vi "MGCC_StaEst_initial_3.vi"() -> ()   [LabVIEW 2016]
uses:
  <vilib>/imath/engines/lvmath2/RunTimeEngine/RunTimeType/NIMS_RunTimeType_From StrictType (excl LVString).vi
  <instcachedir>/0/NIMS_RunTimeType_From StrictType (excl LVString)_BBF44FB49F834B71AF7A14CCEDF8BECD.lvgen/NIMS_RunTimeType_From StrictType (excl LVString)_BBF44FB49F834B71AF7A14CCEDF8BECD_032.vi
  <instcachedir>/0/NIMS_RunTimeType_From StrictType (excl LVString)_BBF44FB49F834B71AF7A14CCEDF8BECD.lvgen/NIMS_RunTimeType_From StrictType (excl LVString)_BBF44FB49F834B71AF7A14CCEDF8BECD_031.vi
  <vilib>/imath/engines/lvmath2/RunTimeEngine/Struct/NIMS_StructSetField.vi
  <vilib>/imath/engines/lvmath2/RunTimeEngine/Struct/NIMS_StructGetField.vi
  <vilib>/imath/engines/lvmath2/RunTimeEngine/RunTimeType/NIMS_RunTimeType_To Numeric.vi
  <instcachedir>/0/NIMS_RunTimeType_To Numeric_19D51BCABB82435A94073491761E42EE.lvgen/NIMS_RunTimeType_To Numeric_19D51BCABB82435A94073491761E42EE_009.vi
  <vilib>/imath/engines/lvmath2/RunTimeEngine/RangeToken/NIMS_Range.vi
  <instcachedir>/0/NIMS_Range_A7C094595B484CA7AF10685B02D808ED.lvgen/NIMS_Range_A7C094595B484CA7AF10685B02D808ED_000.vi
  <instcachedir>/0/NIMS_RunTimeType_From StrictType (excl LVString)_BBF44FB49F834B71AF7A14CCEDF8BECD.lvgen/NIMS_RunTimeType_From StrictType (excl LVString)_BBF44FB49F834B71AF7A14CCEDF8BECD_010.vi
  <vilib>/imathl/engines/lvmath/Functions/Error Handling/Create Error.vi
  <instcachedir>/0/NIMS_RunTimeType_To Numeric_19D51BCABB82435A94073491761E42EE.lvgen/NIMS_RunTimeType_To Numeric_19D51BCABB82435A94073491761E42EE_004.vi
  <instcachedir>/0/NIMS_RunTimeType_From StrictType (excl LVString)_BBF44FB49F834B71AF7A14CCEDF8BECD.lvgen/NIMS_RunTimeType_From StrictType (excl LVString)_BBF44FB49F834B71AF7A14CCEDF8BECD_024.vi
  <instcachedir>/0/NIMS_RunTimeType_To Numeric_19D51BCABB82435A94073491761E42EE.lvgen/NIMS_RunTimeType_To Numeric_19D51BCABB82435A94073491761E42EE_008.vi
  <vilib>/imath/engines/lvmath2/RunTimeEngine/NodeEndStatement/NIMS_NodeEndStatement_Output.vi
  <instcachedir>/0/NIMS_NodeEndStatement_Output_53EC0D466D134D7ABD903AC30B43404B.lvgen/NIMS_NodeEndStatement_Output_53EC0D466D134D7ABD903AC30B43404B_001.vi
  <instcachedir>/0/NIMS_NodeEndStatement_Output_53EC0D466D134D7ABD903AC30B43404B.lvgen/NIMS_NodeEndStatement_Output_53EC0D466D134D7ABD903AC30B43404B_011.vi
  <instcachedir>/0/NIMS_NodeEndStatement_Output_53EC0D466D134D7ABD903AC30B43404B.lvgen/NIMS_NodeEndStatement_Output_53EC0D466D134D7ABD903AC30B43404B_023.vi
  <instcachedir>/0/NIMS_NodeEndStatement_Output_53EC0D466D134D7ABD903AC30B43404B.lvgen/NIMS_NodeEndStatement_Output_53EC0D466D134D7ABD903AC30B43404B_029.vi
  <instcachedir>/0/NIMS_NodeEndStatement_Output_53EC0D466D134D7ABD903AC30B43404B.lvgen/NIMS_NodeEndStatement_Output_53EC0D466D134D7ABD903AC30B43404B_019.vi
  <vilib>/imath/engines/lvmath2/RunTimeEngine/ErrorHandling/NIMS_Finalize Error.vi
panel:
  out "iterMax":i32
  out "tol":dbl
  out "MeaIdx":cluster{"PN":dbl[], "QN":dbl[], "VN":dbl[]}
  out "MeaPha":T1
  out "interleaved array":dbl[](array[numeric])
  out "error out":errorcluster
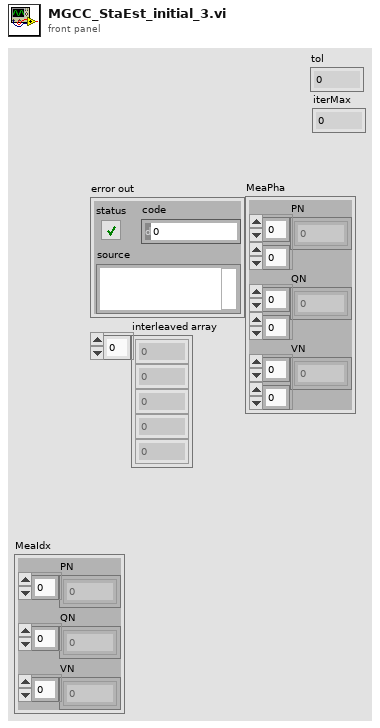
[diagram p1: front panel]
types:
  T1 = cluster{"PN":i32[][], "QN":i32[][], "VN":i32[][]}
  T2 = cluster{"Node":dbl, "Line":dbl, "StateVar":i32, "Zeroinj":i32}
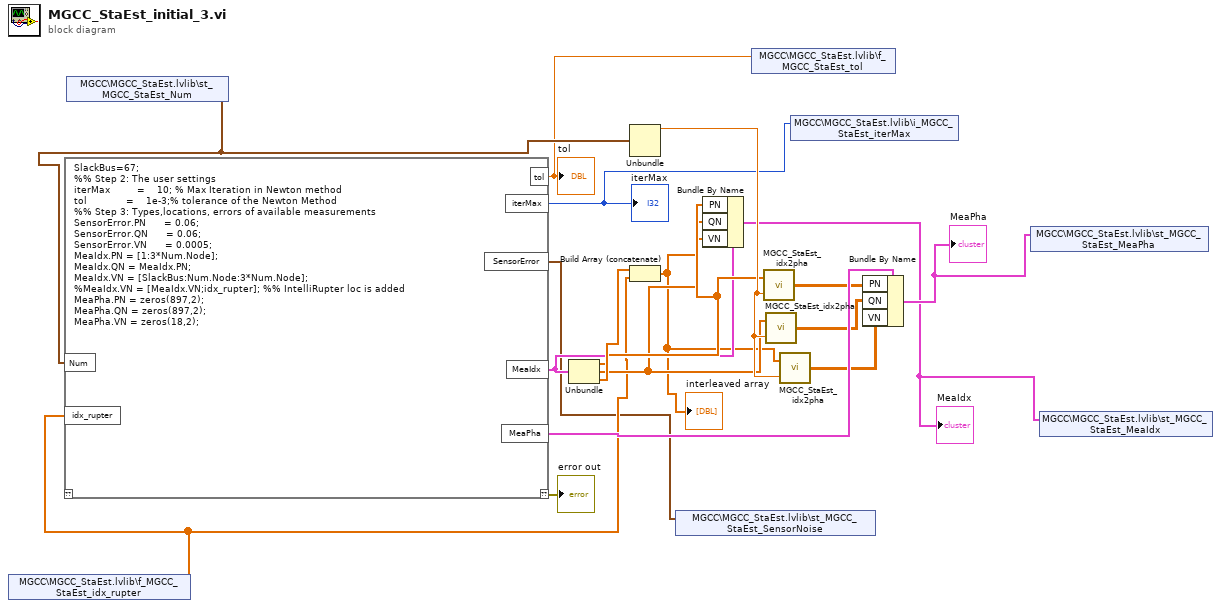
[diagram p0: block diagram]
diagram:
  n1 = shared-variable "MGCC\\MGCC_StaEst.lvlib\\f_MGCC_StaEst_idx_rupter"() -> (w6:dbl[])  [unwired: 1 in, 1 out]
  n2 = shared-variable "MGCC\\MGCC_StaEst.lvlib\\st_MGCC_StaEst_Num"() -> (w7:T2)  [unwired: 1 in, 1 out]
  n3 = mathscript code="SlackBus=67;\n%% Step 2: The user settings\niterMax         =    10; % Max Iteration in Newton method\ntol             =    1e-3;% tolerance of the Newton Method\n%% Step 3: Types,locations, errors of available measurements\nSensorError.PN      = 0.06;\nSensorError.QN      = 0.06;\nSensorError.VN      = 0.0005;\nMeaIdx.PN = [1:3*Num.Node];\nMeaIdx.QN = MeaIdx.PN;\nMeaIdx.VN = [SlackBus:Num.Node:3*Num.Node];\n%MeaIdx.VN = [MeaIdx.VN;idx_rupter]; %% IntelliRupter loc is added\nMeaPha.PN = zeros(897,2);\nMeaPha.QN = zeros(897,2);\nMeaPha.VN = zeros(18,2);"("Num"=w7, "idx_rupter"=w6) -> ("??"=→"error out":errorcluster, "MeaIdx"=w10:cluster{"PN":dbl[], "QN":dbl[], "VN":dbl[]}, "MeaPha"=w15:T1, "SensorError"=w1:cluster{"PN":dbl, "QN":dbl, "VN":dbl}, "iterMax"=w3:i32, "tol"=w2:dbl)  [unwired: 1 in]
  "tol" <- w2
  "iterMax" <- w3
  n4 = Unbundle(w10) -> ("PN"=w11:dbl[], "QN"=w9:dbl[], "VN"=w17:dbl[])
  n5 = Unbundle(w7) -> ("Node"=w16:dbl)  [unwired: 3 out]
  n6 = Build Array (concatenate)(w17, w6) -> (w8:dbl[])
  "interleaved array" <- w8
  n7 = shared-variable "MGCC\\MGCC_StaEst.lvlib\\st_MGCC_StaEst_SensorNoise"(w1) -> ()  [unwired: 1 in, 1 out]
  n8 = Bundle By Name(cluster=w10, "PN"=w11, "QN"=w9, "VN"=w8) -> (w4:cluster{"PN":dbl[], "QN":dbl[], "VN":dbl[]})
  "MeaIdx" <- w4
  n9 = shared-variable "MGCC\\MGCC_StaEst.lvlib\\f_MGCC_StaEst_tol"(w2) -> ()  [unwired: 1 in, 1 out]
  n10 = call "MGCC_StaEst_idx2pha.vi"("n"=w16, "Index"=w11) -> ("byphase"=w14:dbl[][])
  n11 = call "MGCC_StaEst_idx2pha.vi"("n"=w16, "Index"=w9) -> ("byphase"=w13:dbl[][])
  n12 = call "MGCC_StaEst_idx2pha.vi"("n"=w16, "Index"=w8) -> ("byphase"=w12:dbl[][])
  n13 = shared-variable "MGCC\\MGCC_StaEst.lvlib\\i_MGCC_StaEst_iterMax"(w3) -> ()  [unwired: 1 in, 1 out]
  n14 = Bundle By Name(cluster=w15, "PN"=w14, "QN"=w13, "VN"=w12) -> (w5:T1)
  "MeaPha" <- w5
  n15 = shared-variable "MGCC\\MGCC_StaEst.lvlib\\st_MGCC_StaEst_MeaPha"(w5) -> ()  [unwired: 1 in, 1 out]
  n16 = shared-variable "MGCC\\MGCC_StaEst.lvlib\\st_MGCC_StaEst_MeaIdx"(w4) -> ()  [unwired: 1 in, 1 out]
